vi "1553B_CMD_v4.vi"(9 "RT地址":u8, 10 "控制指令子地址(默认：11010":u16=26 format="%.0b", 11 "数据字数组":u16[](array[numeric]) format="%.0x") -> (3 "1553B指令":string)   [LabVIEW 2012]
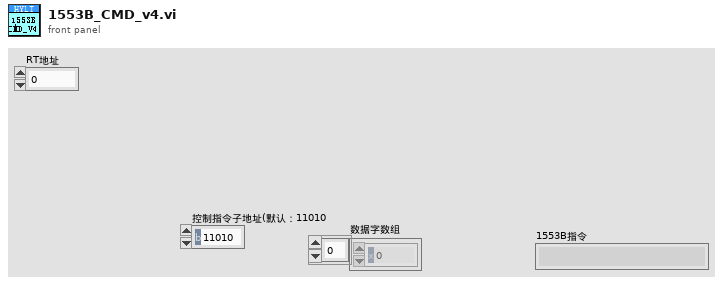
[diagram p1: front panel]
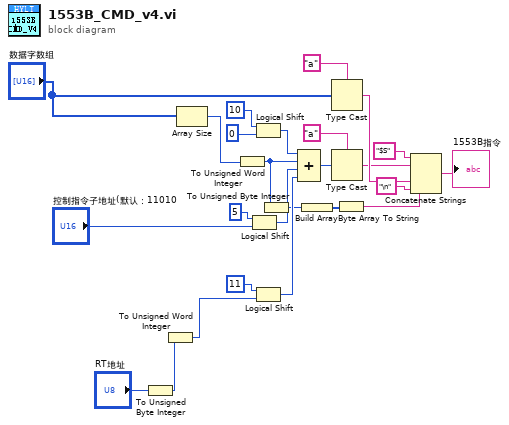
[diagram p0: block diagram]
diagram:
  n1 = To Unsigned Byte Integer(number="RT地址") -> (unsigned 8bit integer=w3:u8)
  n2 = To Unsigned Word Integer(number=w3) -> (unsigned 16bit integer=w2:u16)
  n3 = Array Size(array="数据字数组") -> (size(s)=w15:i32)
  n4 = To Unsigned Word Integer(number=w15) -> (unsigned 16bit integer=w8:u16)
  n5 = Logical Shift(y=i16 5, x="控制指令子地址(默认：11010") -> (x << y=w20:u16)
  n6 = Logical Shift(y=i16 10, x=u16 0) -> (x << y=w22:u16)
  n7 = Logical Shift(y=i16 11, x=w2) -> (x << y=w17:u16)
  n8 = To Unsigned Byte Integer(number=w8) -> (unsigned 8bit integer=w6:u8)
  n9 = Compound Arithmetic op=ADD(w22, w8, w20, w17) -> (w16:u16)
  n10 = Build Array(w6) -> (w7:u8[])
  n11 = Type Cast(type="a" ("类型"), x="数据字数组") -> (*(type *) &x=w13:string)
  n12 = Type Cast(type="a" ("类型"), x=w16) -> (*(type *) &x=w12:string)
  n13 = Byte Array To String(unsigned byte array=w7) -> (string=w5:string)
  n14 = Concatenate Strings("$S" ("字符串"), w12, w5, w13, "\n" ("字符串")) -> (→"1553B指令":string)
